vi "Periodic Tasks.vi"(8 "error in":errorcluster) -> ()   [LabVIEW 2019]
doc: "This VI runs in parallel to other tasks. It can contain as many user-defined periodic loops as you need. These can carry out PID or other sorts of timed response."
uses:
  <vilib>/Rock Robotics/Network Tables/NT Read Boolean.vi
  <vilib>/Rock Robotics/Network Tables/NT Write Number.vi
  <vilib>/Rock Robotics/Network Tables/NT Read Number.vi
  <vilib>/Rock Robotics/Network Tables/NT Write Boolean.vi
  <vilib>/Rock Robotics/WPI/Utilities/WPI_GetSetVariantRefNum.vi
  <vilib>/Rock Robotics/Network Tables/NT Write Numeric Array.vi
  <vilib>/Rock Robotics/WPI/RobotDrive/WPI_RobotDriveArcadeDrive_Standard(NoSaturation).vi
  <vilib>/express/express arith-compare/Formula/XNode/ExpressFormulaBlockNode.xnode
  <vilib>/Rock Robotics/Network Tables/NT Write String.vi
  <vilib>/Rock Robotics/Network Tables/NT Read String.vi
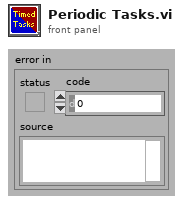
[diagram p1: front panel]
types:
  T1 = typedef "WPI_JoystickDevRef.ctl" = cluster{"Device":T2}
  T2 = typedef "WPI_JoystickDeviceEnum.ctl" = enum16{"USB 0", "USB 1", "USB 2", "USB 3", "USB 4", "USB 5"}
  T3 = typedef "WPI_RobotDriveDevRef.ctl" = cluster{"DevStatus":errorcluster, "Motors[]":T4[], "Square Inputs":bool, "Max Output":dbl}
  T4 = typedef "WPI_MotorControlDeviceRef.ctl" = cluster{"DeviceStatus":errorcluster, "Type":T5, "PWM":cluster{"PWM Channel":T6, "DeadBand":T7}, "CAN":cluster{"Device Number":u8, "SetOutput VI Ref":variant, "GetOutput VI Ref":variant, "Enable VI Ref":variant, "Disable VI Ref":variant, "Data":variant}, "Invert":bool, "DIO PWM":cluster{"PWM \"Enable\" Channel":T6, "DIOChannel":T8, "PWM Rate":dbl}}
  T5 = typedef "WPI_MotorControlType.ctl" = enum16{"PWM", "CAN", "DIO PWM"}
  T6 = typedef "FPGA_DIOPWMChannel.ctl" = enum8{"PWM 0", "PWM 1", "PWM 2", "PWM 3", "PWM 4", "PWM 5", "PWM 6", "PWM 7", "PWM 8", "PWM 9", "PWM MXP 0", "PWM MXP 1", "PWM MXP 2", "PWM MXP 3", "PWM MXP 4", "PWM MXP 5", "PWM MXP 6", "PWM MXP 7", "PWM MXP 8", "PWM MXP 9", "Invalid"}
  T7 = typedef "WPI_PWMDeadband.ctl" = cluster{"Name":string, "maxPositivePwm":i32, "minPositivePwm":i32, "centerPwm":i32, "maxNegativePwm":i32, "minNegativePwm":i32, "angularRange":u16}
  T8 = typedef "FPGA_DIOChannel.ctl" = enum8{"DIO 0", "DIO 1", "DIO 2", "DIO 3", "DIO 4", "DIO 5", "DIO 6", "DIO 7", "DIO 8", "DIO 9", "DIO MXP 0", "DIO MXP 1", "DIO MXP 2", "DIO MXP 3", "DIO MXP 4", "DIO MXP 5", "DIO MXP 6", "DIO MXP 7", "DIO MXP 8", "DIO MXP 9", "DIO MXP 10", "DIO MXP 11", "DIO MXP 12", "DIO MXP 13", "DIO MXP 14", "DIO MXP 15", "SPI Port CS1", "SPI Port CS2", "SPI Port CS3", "SPI Port MISO", "SPI Port MOSI", "Invalid"}
  T9 = cluster{"JoystickDevRef":T1, "RobotDriveDevRef":T3}
  T10 = typedef "Color Sensor V3 DevRef.ctl" = cluster{"I2CDevRef":T11}
  T11 = typedef "WPI_I2CDevRef.ctl" = cluster{"DevStatus":errorcluster, "Device Address":u8, "Handle":i32, "I2C Bus":T12}
  T12 = typedef "i2c_bus.ctl" = enum16{"I2C On-Board", "I2C MXP", "Invalid"}
  T13 = typedef "WPI_SwitchDevRef.ctl" = cluster{"DevStatus":errorcluster, "DIO Channel":T8, "CntIndex":T14, "Normally Closed":bool}
  T14 = typedef "FPGA_CounterCtrSystemIndex.ctl" = enum8{"Ctr 0", "Ctr 1", "Ctr 2", "Ctr 3", "Ctr 4", "Ctr 5", "Ctr 6", "Ctr 7", "Invalid"}
  T15 = typedef "WPI_ServoDeviceRef.ctl" = cluster{"DeviceStatus":errorcluster, "PWM Channel":T6, "DeadBand":T7}
  T16 = typedef "WPI_EncoderDevRef.ctl" = cluster{"DevStatus":errorcluster, "EncoderIndex":T17, "CounterIndex":T14, "DistancePerCount":dbl, "Decoding Type":T18}
  T17 = typedef "FPGA_EncoderIdx.ctl" = enum8{"Enc 0", "Enc 1", "Enc 2", "Enc 3", "Enc 4", "Enc 5", "Enc 6", "Enc 7", "Invalid"}
  T18 = typedef "WPI_EncoderType.ctl" = enum16{"1x", "2x", "4x"}
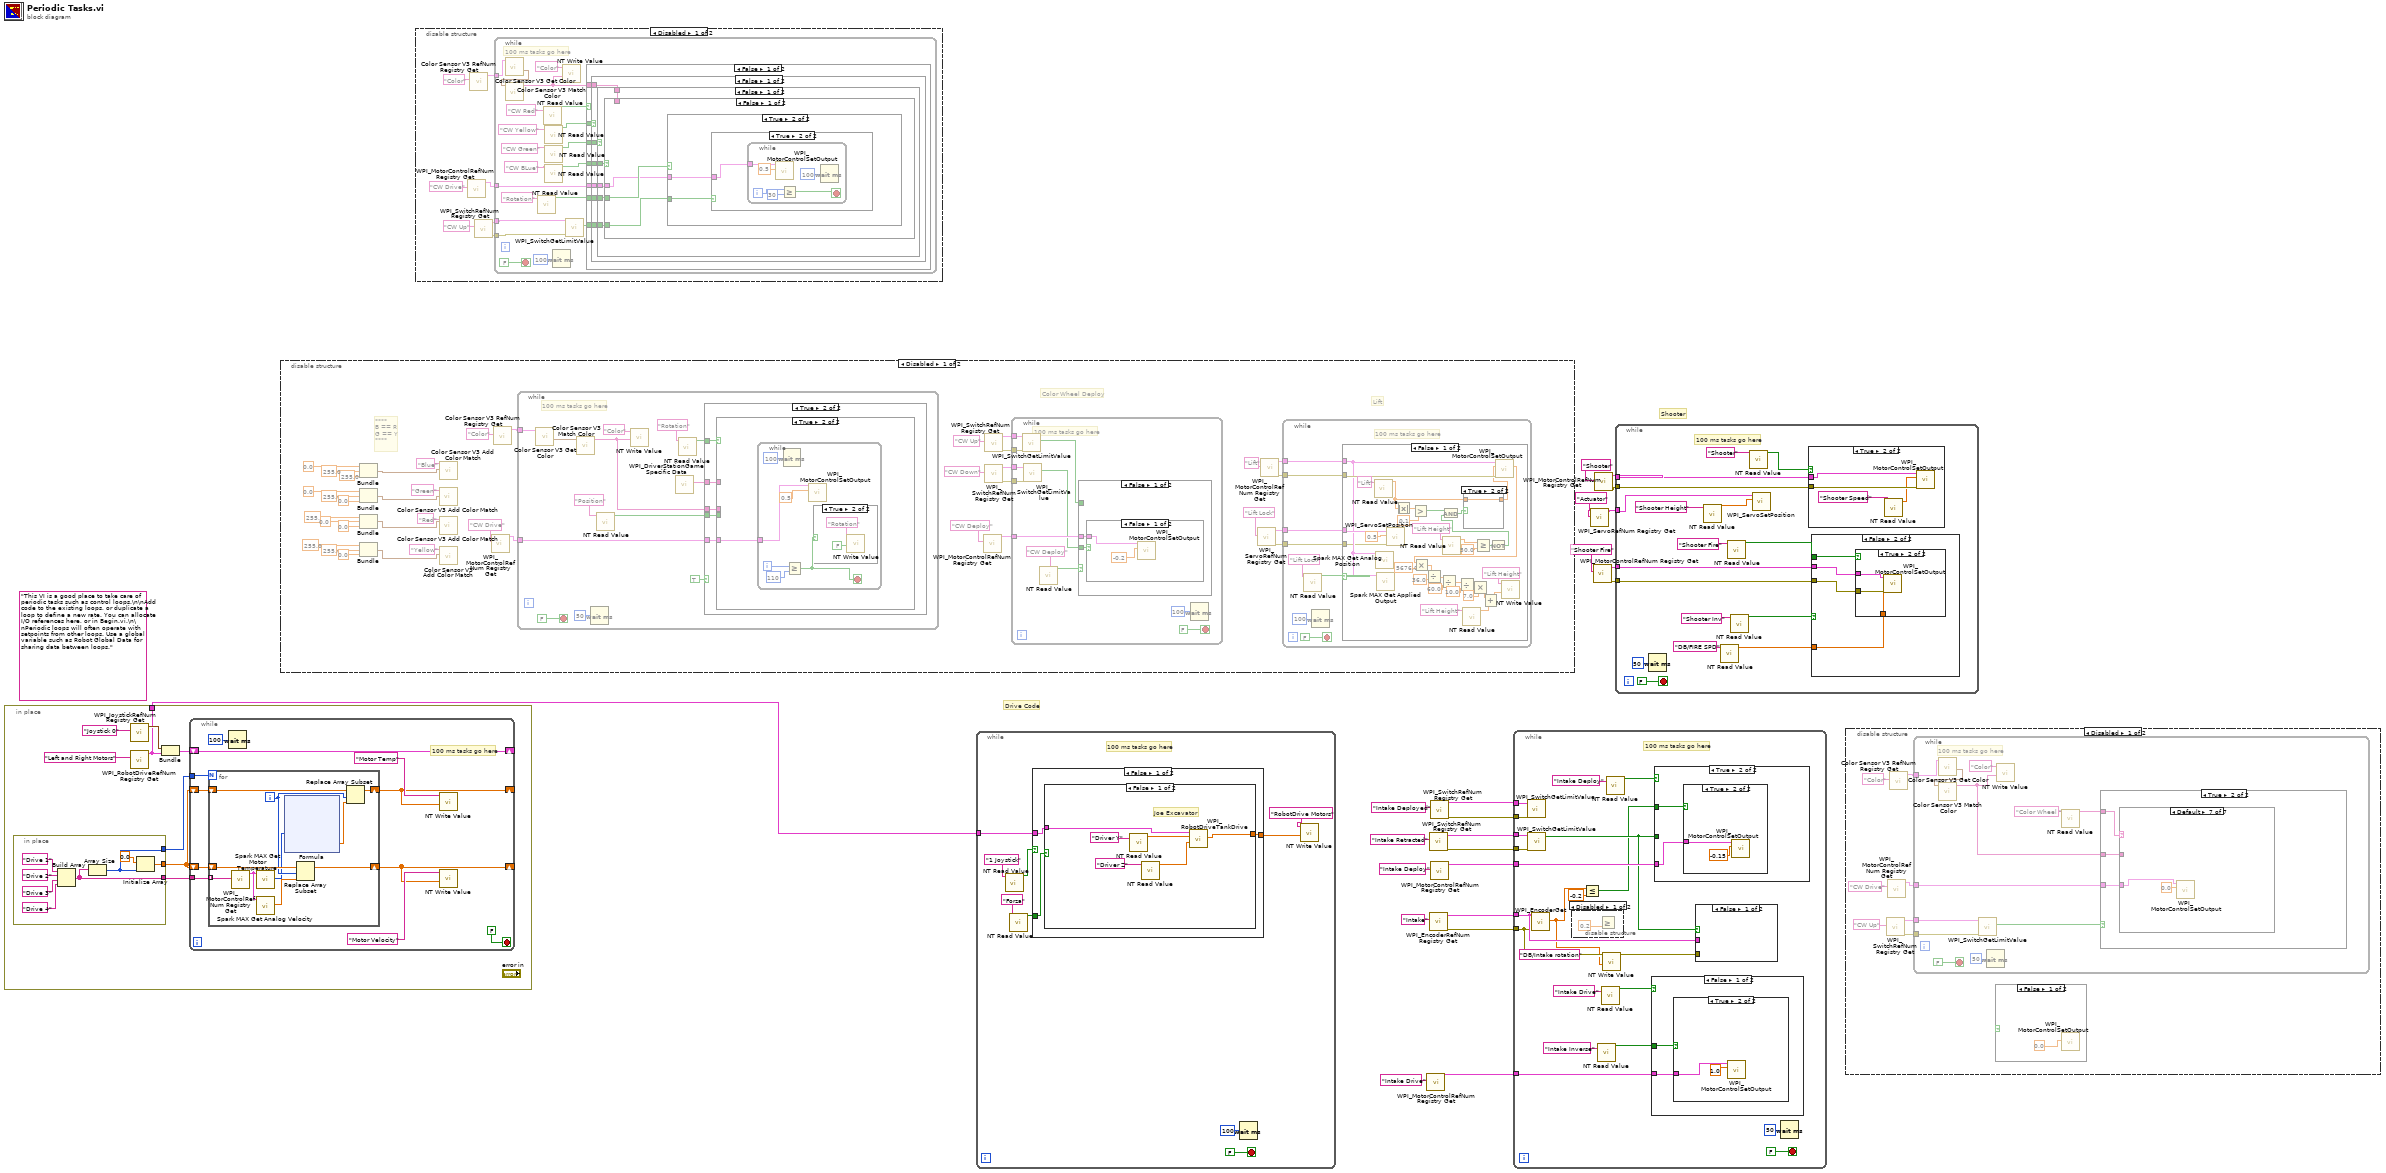
[diagram p0: block diagram]
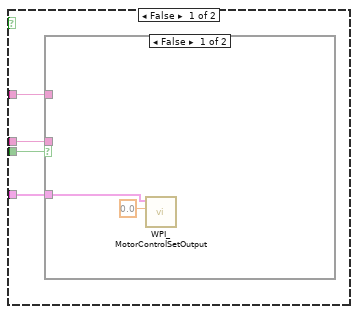
[diagram p3: hidden frame]
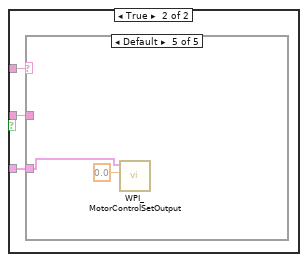
[diagram p4: hidden frame]
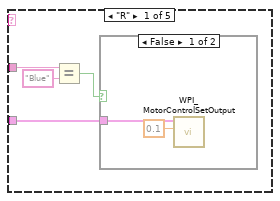
[diagram p5: hidden frame]
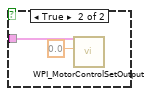
[diagram p6: hidden frame]
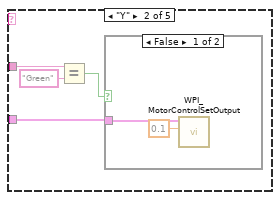
[diagram p7: hidden frame]
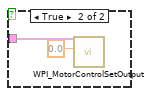
[diagram p8: hidden frame]
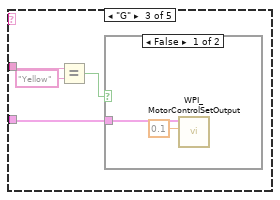
[diagram p9: hidden frame]
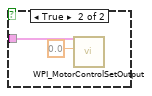
[diagram p10: hidden frame]
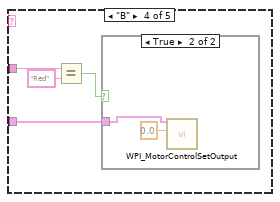
[diagram p11: hidden frame]
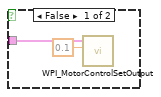
[diagram p12: hidden frame]
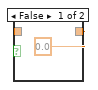
[diagram p14: hidden frame]
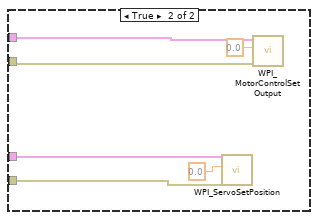
[diagram p15: hidden frame]
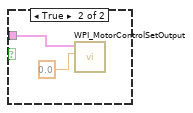
[diagram p16: hidden frame]
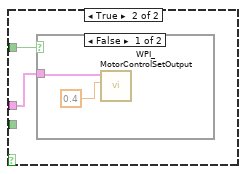
[diagram p17: hidden frame]
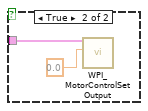
[diagram p18: hidden frame]
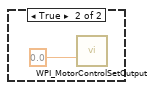
[diagram p20: hidden frame]
diagram:
  (unwired) "This VI is a good place to take care of periodic tasks such as control loops.\n\nAdd code to the existing loops, or duplicate a loop to define a new rate. You can allocate I/O references here, or in Begin.vi.\n\nPeriodic loops will often operate with setpoints from other loops. Use a global variable such as Robot Global Data for sharing data between loops."
  # "Shooter"
  # "Drive Code"
  n1 = in-place {
    in-place-border: [w23] -> w1
    n2 = in-place {
      in-place-border: [w34] -> w26
      in-place-border: [w33] -> w25
      in-place-border: [w31] -> w24
      n3 = Build Array("Drive 1", "Drive 2", "Drive 3", "Drive 4") -> (w34:string[])
      n4 = Array Size(array=w34) -> (size(s)=w33:i32)
      n5 = Initialize Array(0.0 ("element"), w33) -> (w31:dbl[])
    }
    n6 = call <vilib>:"WPI_JoystickRefNum Registry Get.vi"("refnum name"="Joystick 0") -> ("JoystickDevRef"=w28:T1)  [unwired: 1 in, 9 out]
    n7 = call <vilib>:"WPI_RobotDriveRefNum Registry Get.vi"("refnum name"="Left and Right Motors") -> ("RobotDriveDevRef"=w23:T3)  [unwired: 1 in, 9 out]
    n8 = Bundle("JoystickDevRef"=w28, "RobotDriveDevRef"=w23) -> (w27:T9)  [unwired: 1 out]
    n9 = while {
      shift-right: [w47] -> _
      shift-left: w27 -> [w47]
      tunnel: w26 -> [w44]
      tunnel: w25 -> [w43]
      shift-right: [w39] -> _
      shift-left: w24 -> [w42]
      shift-right: [w40] -> _
      shift-left: w24 -> [w41]
      stop <- FALSE stop-if-true
      # "100 ms tasks go here"
      n10 = for {
        N: w43 -> [_]
        tunnel: w44 -> [w58] mode=indexing
        shift-right: [w55] -> w40
        shift-left: w41 -> [w56]
        shift-right: [w53] -> w39
        shift-left: w42 -> [w57]
        i -> [w52]
        n11 = call <vilib>:"WPI_MotorControlRefNum Registry Get.vi"("refnum name"=w58) -> ("MotorControlDevRef"=w59:T4)  [unwired: 9 in, 1 out]
        n12 = call <vilib>:"Spark MAX Get Motor Temperature.vi"("MotorControlDevRef in"=w59) -> ("Motor Temperature"=w51:u8)  [unwired: 7 in, 3 out]
        n13 = call <vilib>:"Spark MAX Get Analog Velocity.vi"("MotorControlDevRef in"=w59) -> ("Analog Velocity"=w54:dbl)  [unwired: 7 in, 3 out]
        n14 = xnode "Formula"("degC"=w51) -> ("Result"=w50:dbl)  [unwired: 1 in, 1 out]
        n15 = Replace Array Subset(array=w56, new element=w54, index=w52) -> (w55:dbl[])
        n16 = Replace Array Subset(array=w57, new element=w50, index=w52) -> (w53:dbl[])
      }
      n17 = Wait (ms)(milliseconds to wait=u32 100) -> ()  [unwired: 1 out]
      n18 = call-poly <vilib>:"NT Write Value.vi"("Numeric Array"=w39, "Name"="Motor Temp") -> ()  [unwired: 9 in, 1 out]
      n19 = call-poly <vilib>:"NT Write Value.vi"("Numeric Array"=w40, "Name"="Motor Velocity") -> ()  [unwired: 9 in, 1 out]
    }
  }
  n20 = disable-structure shown="Disabled" {
    frame Disabled {
      # "Lift"
      # "****\nB == R\nG == Y\n****"
      # "Color Wheel Deploy"
      n21 = Bundle(0.0, 255.0, 255.0) -> (w99:cluster{dbl, dbl, dbl})  [unwired: 1 in]
      n22 = Bundle(0.0, 255.0, 0.0) -> (w94:cluster{dbl, dbl, dbl})  [unwired: 1 in]
      n23 = Bundle(255.0, 0.0, 0.0) -> (w87:cluster{dbl, dbl, dbl})  [unwired: 1 in]
      n24 = Bundle(255.0, 255.0, 0.0) -> (w86:cluster{dbl, dbl, dbl})  [unwired: 1 in]
      n25 = call <vilib>:"Color Sensor V3 Add Color Match.vi"("Color"=w94, "Name"="Green") -> ()  [unwired: 10 in]
      n26 = call <vilib>:"Color Sensor V3 Add Color Match.vi"("Color"=w87, "Name"="Red") -> ()  [unwired: 10 in]
      n27 = call <vilib>:"Color Sensor V3 Add Color Match.vi"("Color"=w99, "Name"="Blue") -> ()  [unwired: 10 in]
      n28 = call <vilib>:"Color Sensor V3 Add Color Match.vi"("Color"=w86, "Name"="Yellow") -> ()  [unwired: 10 in]
      n29 = call <vilib>:"WPI_MotorControlRefNum Registry Get.vi"("refnum name"="CW Drive") -> ("MotorControlDevRef"=w68:T4)  [unwired: 9 in, 1 out]
      n30 = call <vilib>:"Color Sensor V3 RefNum Registry Get.vi"("refnum name"="Color") -> ("ColorSensorDevRef"=w70:T10)  [unwired: 9 in, 1 out]
      n31 = while {
        tunnel: w70 -> [w116]
        tunnel: w68 -> [w112]
        stop <- FALSE stop-if-true
        # "100 ms tasks go here"
        n32 = call <vilib>:"Color Sensor V3 Get Color.vi"("ColorSensorDevRef"=w116) -> ("Normalized Color"=w115:cluster{"R":dbl, "G":dbl, "B":dbl})  [unwired: 7 in, 3 out]
        n33 = call <vilib>:"Color Sensor V3 Match Color.vi"("Measured Color"=w115) -> ("Matched Color Name"=w113:string)  [unwired: 8 in, 2 out]
        n34 = Wait (ms)(milliseconds to wait=u32 50) -> ()  [unwired: 1 out]
        n35 = call-poly <vilib>:"NT Read Value.vi"("Name"="Position") -> ("Boolean"=w106:bool)  [unwired: 9 in, 1 out]
        n36 = call-poly <vilib>:"NT Write Value.vi"("String"=w113, "Name"="Color") -> ()  [unwired: 9 in, 1 out]
        n37 = call <vilib>:"WPI_DriverStationGame Specific Data.vi"() -> ("Game Specific Data"=w111:string)  [unwired: 11 in]
        n38 = call-poly <vilib>:"NT Read Value.vi"("Name"="Rotation") -> ("Boolean"=w109:bool)  [unwired: 9 in, 1 out]
        n39 = case shown="True" TRUE {
          tunnel: w111 -> [_ w122]
          tunnel: w113 -> [_ w121]
          tunnel: w112 -> [_ w120]
          tunnel: w109 -> [_ w123]
          tunnel: w106 -> [_ w119]
          frame False {
          }
          frame True {
            n40 = case shown="True" w123 {
              tunnel: w122 -> [w127 _]
              tunnel: w121 -> [w126 _]
              tunnel: w120 -> [w125 w167]
              tunnel: w119 -> [w124 _]
              frame False {
                n41 = case shown="False" w124 {
                  tunnel: w127 -> [_ w132]
                  tunnel: w126 -> [_ w131]
                  tunnel: w125 -> [w128 w130]
                  frame False {
                    n42 = call <vilib>:"WPI_MotorControlSetOutput.vi"("Output"=0.0, "MotorControlDevRef"=w128) -> ()  [unwired: 7 in, 3 out]
                  }
                  frame True {
                    n43 = case shown="Default" w132 {
                      tunnel: w131 -> [w136 w141 w150 w158 _]
                      tunnel: w130 -> [w134 w142 w149 w157 w165]
                      frame "R" {
                        n44 = Equal?(x=w136, y="Blue") -> (x = y?=w135:bool)
                        n45 = case shown="False" w135 {
                          tunnel: w134 -> [w138 w140]
                          frame False {
                            n46 = call <vilib>:"WPI_MotorControlSetOutput.vi"("Output"=0.1, "MotorControlDevRef"=w138) -> ()  [unwired: 7 in, 3 out]
                          }
                          frame True {
                            n47 = call <vilib>:"WPI_MotorControlSetOutput.vi"("Output"=0.0, "MotorControlDevRef"=w140) -> ()  [unwired: 7 in, 3 out]
                          }
                        }
                      }
                      frame "Y" {
                        n48 = Equal?(x=w141, y="Green") -> (x = y?=w144:bool)
                        n49 = case shown="False" w144 {
                          tunnel: w142 -> [w146 w148]
                          frame False {
                            n50 = call <vilib>:"WPI_MotorControlSetOutput.vi"("Output"=0.1, "MotorControlDevRef"=w146) -> ()  [unwired: 7 in, 3 out]
                          }
                          frame True {
                            n51 = call <vilib>:"WPI_MotorControlSetOutput.vi"("Output"=0.0, "MotorControlDevRef"=w148) -> ()  [unwired: 7 in, 3 out]
                          }
                        }
                      }
                      frame "G" {
                        n52 = Equal?(x=w150, y="Yellow") -> (x = y?=w152:bool)
                        n53 = case shown="False" w152 {
                          tunnel: w149 -> [w154 w156]
                          frame False {
                            n54 = call <vilib>:"WPI_MotorControlSetOutput.vi"("Output"=0.1, "MotorControlDevRef"=w154) -> ()  [unwired: 7 in, 3 out]
                          }
                          frame True {
                            n55 = call <vilib>:"WPI_MotorControlSetOutput.vi"("Output"=0.0, "MotorControlDevRef"=w156) -> ()  [unwired: 7 in, 3 out]
                          }
                        }
                      }
                      frame "B" {
                        n56 = Equal?(x=w158, y="Red") -> (x = y?=w160:bool)
                        n57 = case shown="True" w160 {
                          tunnel: w157 -> [w161 w163]
                          frame False {
                            n58 = call <vilib>:"WPI_MotorControlSetOutput.vi"("Output"=0.1, "MotorControlDevRef"=w161) -> ()  [unwired: 7 in, 3 out]
                          }
                          frame True {
                            n59 = call <vilib>:"WPI_MotorControlSetOutput.vi"("Output"=0.0, "MotorControlDevRef"=w163) -> ()  [unwired: 7 in, 3 out]
                          }
                        }
                      }
                      frame Default {
                        n60 = call <vilib>:"WPI_MotorControlSetOutput.vi"("Output"=0.0, "MotorControlDevRef"=w165) -> ()  [unwired: 7 in, 3 out]
                      }
                    }
                  }
                }
              }
              frame True {
                n61 = while {
                  tunnel: w167 -> [w168]
                  i -> [w172]
                  stop <- w170 stop-if-true
                  n62 = Wait (ms)(milliseconds to wait=u32 100) -> ()  [unwired: 1 out]
                  n63 = Greater Or Equal?(x=w172, y=110) -> (x >= y?=w170:bool)
                  n64 = call <vilib>:"WPI_MotorControlSetOutput.vi"("Output"=0.5, "MotorControlDevRef"=w168) -> ()  [unwired: 7 in, 3 out]
                  n65 = case shown="True" w170 {
                    frame False {
                    }
                    frame True {
                      n66 = call-poly <vilib>:"NT Write Value.vi"("Boolean"=FALSE, "Name"="Rotation") -> ()  [unwired: 9 in, 1 out]
                    }
                  }
                }
              }
            }
          }
        }
      }
      n67 = call <vilib>:"WPI_MotorControlRefNum Registry Get.vi"("refnum name"="CW Deploy") -> ("MotorControlDevRef"=w82:T4)  [unwired: 9 in, 1 out]
      n68 = call <vilib>:"WPI_SwitchRefNum Registry Get.vi"("refnum name"="CW Up") -> ("error out"=w74:errorcluster, "SwitchDevRef"=w73:T13)  [unwired: 9 in]
      n69 = call <vilib>:"WPI_SwitchRefNum Registry Get.vi"("refnum name"="CW Down") -> ("error out"=w76:errorcluster, "SwitchDevRef"=w75:T13)  [unwired: 9 in]
      n70 = while {
        tunnel: w82 -> [w230]
        tunnel: w76 -> [w229]
        tunnel: w75 -> [w228]
        tunnel: w74 -> [w226]
        tunnel: w73 -> [w225]
        stop <- FALSE stop-if-true
        # "100 ms tasks go here"
        n71 = call <vilib>:"WPI_SwitchGetLimitValue.vi"("error in (no error)"=w226, "SwitchDevRef"=w225) -> ("Switch Pressed"=w224:bool)  [unwired: 7 in, 2 out]
        n72 = call <vilib>:"WPI_SwitchGetLimitValue.vi"("error in (no error)"=w229, "SwitchDevRef"=w228) -> ("Switch Pressed"=w227:bool)  [unwired: 7 in, 2 out]
        n73 = call-poly <vilib>:"NT Read Value.vi"("Name"="CW Deploy") -> ("Boolean"=w231:bool)  [unwired: 9 in, 1 out]
        n74 = case shown="False" w231 {
          tunnel: w230 -> [w236 w241]
          tunnel: w227 -> [w235 _]
          tunnel: w224 -> [_ w242]
          frame False {
            n75 = case shown="False" w235 {
              tunnel: w236 -> [w237 w240]
              frame False {
                n76 = call <vilib>:"WPI_MotorControlSetOutput.vi"("Output"=-0.2 ("Motor Output"), "MotorControlDevRef"=w237) -> ()  [unwired: 7 in, 3 out]
              }
              frame True {
                n77 = call <vilib>:"WPI_MotorControlSetOutput.vi"("Output"=0.0 ("Motor Output"), "MotorControlDevRef"=w240) -> ()  [unwired: 7 in, 3 out]
              }
            }
          }
          frame True {
            n78 = case shown="False" w242 {
              tunnel: w241 -> [w243 w246]
              frame False {
                n79 = call <vilib>:"WPI_MotorControlSetOutput.vi"("Output"=0.4 ("Motor Output"), "MotorControlDevRef"=w243) -> ()  [unwired: 7 in, 3 out]
              }
              frame True {
                n80 = call <vilib>:"WPI_MotorControlSetOutput.vi"("Output"=0.0 ("Motor Output"), "MotorControlDevRef"=w246) -> ()  [unwired: 7 in, 3 out]
              }
            }
          }
        }
        n81 = Wait (ms)(milliseconds to wait=u32 100) -> ()  [unwired: 1 out]
      }
      n82 = call <vilib>:"WPI_ServoRefNum Registry Get.vi"("refnum name"="Lift Lock") -> ("error out"=w72:errorcluster, "ServoDeviceRef"=w77:T15)  [unwired: 9 in]
      n83 = call <vilib>:"WPI_MotorControlRefNum Registry Get.vi"("refnum name"="Lift") -> ("error out"=w79:errorcluster, "MotorControlDevRef"=w80:T4)  [unwired: 9 in]
      n84 = while {
        tunnel: w80 -> [w176]
        tunnel: w79 -> [w177]
        tunnel: w77 -> [w181]
        tunnel: w72 -> [w178]
        stop <- FALSE stop-if-true
        # "100 ms tasks go here"
        n85 = call-poly <vilib>:"NT Read Value.vi"("Name"="Lift Lock") -> ("Boolean"=w179:bool)  [unwired: 9 in, 1 out]
        n86 = Wait (ms)(milliseconds to wait=u32 100) -> ()  [unwired: 1 out]
        n87 = case shown="False" w179 {
          tunnel: w181 -> [w215 w223]
          tunnel: w178 -> [w204 w222]
          tunnel: w177 -> [w213 w219]
          tunnel: w176 -> [w207 w220]
          frame False {
            n88 = call-poly <vilib>:"NT Read Value.vi"("Name"="Lift") -> ("Numeric"=w208:dbl)  [unwired: 9 in, 1 out]
            n89 = call <vilib>:"Spark MAX Get Analog Position.vi"("MotorControlDevRef in"=w207) -> ()  [unwired: 7 in, 4 out]
            n90 = call <vilib>:"Spark MAX Get Applied Output.vi"("MotorControlDevRef in"=w207) -> ()  [unwired: 7 in, 4 out]
            n91 = call <vilib>:"WPI_ServoSetPosition.vi"("error in (no error)"=w204, "Position"=0.5, "ServoDeviceRef"=w215) -> ()  [unwired: 7 in, 2 out]
            n92 = Absolute Value(x=w208) -> (abs(x)=w211:dbl)
            n93 = Greater?(x=w211, y=0.1) -> (0:w187:bool)
            n94 = call-poly <vilib>:"NT Read Value.vi"("Name"="Lift Height") -> ("Numeric"=w189:dbl)  [unwired: 9 in, 1 out]
            n95 = call-poly <vilib>:"NT Read Value.vi"("Name"="Lift Height") -> ("Numeric"=w192:dbl)  [unwired: 9 in, 1 out]
            n96 = Greater Or Equal?(x=w189, y=50.0) -> (x >= y?=w185:bool)
            n97 = Not(x=w185) -> (.not. x?=w184:bool)
            n98 = And(x=w187, y=w184) -> (x .and. y?=w186:bool)
            n99 = case shown="True" w186 {
              tunnel: [0.0 w217] -> w209
              tunnel: w208 -> [_ w217]
              frame False {
              }
              frame True {
              }
            }
            n100 = call <vilib>:"WPI_MotorControlSetOutput.vi"("error in (no error)"=w213, "Output"=w209, "MotorControlDevRef"=w207) -> ("Motor Output"=w196:dbl)  [unwired: 6 in, 2 out]
            n101 = Multiply(x=w196, y=5676.0) -> (x*y=w198:dbl)
            n102 = Divide(x=w198, y=36.0) -> (x/y=w201:dbl)
            n103 = Divide(x=w201, y=60.0) -> (x/y=w202:dbl)
            n104 = Divide(x=w202, y=10.0) -> (x/y=w200:dbl)
            n105 = Multiply(x=w200, y=7.0) -> (x*y=w191:dbl)
            n106 = Add(x=w191, y=w192) -> (x+y=w193:dbl)
            n107 = call-poly <vilib>:"NT Write Value.vi"("Numeric"=w193, "Name"="Lift Height") -> ()  [unwired: 9 in, 1 out]
          }
          frame True {
            n108 = call <vilib>:"WPI_ServoSetPosition.vi"("error in (no error)"=w222, "Position"=0.0, "ServoDeviceRef"=w223) -> ()  [unwired: 7 in, 2 out]
            n109 = call <vilib>:"WPI_MotorControlSetOutput.vi"("error in (no error)"=w219, "Output"=0.0, "MotorControlDevRef"=w220) -> ()  [unwired: 6 in, 3 out]
          }
        }
      }
    }
    frame Enabled {
    }
  }
  n110 = disable-structure shown="Disabled" {
    frame Disabled {
      n111 = call <vilib>:"WPI_MotorControlRefNum Registry Get.vi"("refnum name"="CW Drive") -> ("MotorControlDevRef"=w250:T4)  [unwired: 9 in, 1 out]
      n112 = call <vilib>:"Color Sensor V3 RefNum Registry Get.vi"("refnum name"="Color") -> ("ColorSensorDevRef"=w252:T10)  [unwired: 9 in, 1 out]
      n113 = call <vilib>:"WPI_SwitchRefNum Registry Get.vi"("refnum name"="CW Up") -> ("error out"=w247:errorcluster, "SwitchDevRef"=w248:T13)  [unwired: 9 in]
      n114 = while {
        tunnel: w252 -> [w271]
        tunnel: w250 -> [w261]
        tunnel: w248 -> [w258]
        tunnel: w247 -> [w257]
        stop <- FALSE stop-if-true
        # "100 ms tasks go here"
        n115 = call <vilib>:"Color Sensor V3 Get Color.vi"("ColorSensorDevRef"=w271) -> ("Normalized Color"=w270:cluster{"R":dbl, "G":dbl, "B":dbl})  [unwired: 7 in, 3 out]
        n116 = call <vilib>:"Color Sensor V3 Match Color.vi"("Measured Color"=w270) -> ("Matched Color Name"=w255:string)  [unwired: 8 in, 2 out]
        n117 = call-poly <vilib>:"NT Read Value.vi"("Name"="Rotation") -> ("Boolean"=w259:bool)  [unwired: 9 in, 1 out]
        n118 = call-poly <vilib>:"NT Read Value.vi"("Name"="CW Red") -> ("Boolean"=w266:bool)  [unwired: 9 in, 1 out]
        n119 = call-poly <vilib>:"NT Read Value.vi"("Name"="CW Yellow") -> ("Boolean"=w265:bool)  [unwired: 9 in, 1 out]
        n120 = call-poly <vilib>:"NT Read Value.vi"("Name"="CW BLue") -> ("Boolean"=w262:bool)  [unwired: 9 in, 1 out]
        n121 = call-poly <vilib>:"NT Read Value.vi"("Name"="CW Green") -> ("Boolean"=w264:bool)  [unwired: 9 in, 1 out]
        n122 = Wait (ms)(milliseconds to wait=u32 100) -> ()  [unwired: 1 out]
        n123 = call-poly <vilib>:"NT Write Value.vi"("String"=w255, "Name"="Color") -> ()  [unwired: 9 in, 1 out]
        n124 = call <vilib>:"WPI_SwitchGetLimitValue.vi"("error in (no error)"=w257, "SwitchDevRef"=w258) -> ("Switch Pressed"=w256:bool)  [unwired: 7 in, 2 out]
        n125 = case shown="False" w266 {
          tunnel: w265 -> [w280 _]
          tunnel: w264 -> [w279 _]
          tunnel: w262 -> [w278 _]
          tunnel: w255 -> [w277 w334]
          tunnel: w261 -> [w276 w332]
          tunnel: w259 -> [w275 _]
          tunnel: w256 -> [w274 _]
          frame False {
            n126 = case shown="False" w280 {
              tunnel: w279 -> [w286 _]
              tunnel: w278 -> [w285 _]
              tunnel: w277 -> [w284 w327]
              tunnel: w276 -> [w283 w324]
              tunnel: w275 -> [w282 _]
              tunnel: w274 -> [w281 _]
              frame False {
                n127 = case shown="False" w286 {
                  tunnel: w285 -> [w291 _]
                  tunnel: w284 -> [w290 w319]
                  tunnel: w283 -> [w289 w316]
                  tunnel: w282 -> [w288 _]
                  tunnel: w281 -> [w287 _]
                  frame False {
                    n128 = case shown="False" w291 {
                      tunnel: w290 -> [_ w309]
                      tunnel: w289 -> [w293 w308]
                      tunnel: w288 -> [w294 _]
                      tunnel: w287 -> [w292 _]
                      frame False {
                        n129 = case shown="True" w294 {
                          tunnel: w293 -> [w295 w298]
                          tunnel: w292 -> [_ w297]
                          frame False {
                            n130 = call <vilib>:"WPI_MotorControlSetOutput.vi"("Output"=0.0, "MotorControlDevRef"=w295) -> ()  [unwired: 7 in, 3 out]
                          }
                          frame True {
                            n131 = case shown="True" w297 {
                              tunnel: w298 -> [w299 w301]
                              frame False {
                                n132 = call <vilib>:"WPI_MotorControlSetOutput.vi"("Output"=0.0, "MotorControlDevRef"=w299) -> ()  [unwired: 7 in, 3 out]
                              }
                              frame True {
                                n133 = while {
                                tunnel: w301 -> [w306]
                                i -> [w304]
                                stop <- w302 stop-if-true
                                n134 = call <vilib>:"WPI_MotorControlSetOutput.vi"("Output"=0.5, "MotorControlDevRef"=w306) -> ()  [unwired: 7 in, 3 out]
                                n135 = Greater Or Equal?(x=w304, y=30) -> (x >= y?=w302:bool)
                                n136 = Wait (ms)(milliseconds to wait=u32 100) -> ()  [unwired: 1 out]
                                }
                              }
                            }
                          }
                        }
                      }
                      frame True {
                        n137 = Equal?(x=w309, y="Red") -> (x = y?=w310:bool)
                        n138 = case shown="False" w310 {
                          tunnel: w308 -> [w312 w314]
                          frame False {
                            n139 = call <vilib>:"WPI_MotorControlSetOutput.vi"("Output"=0.1, "MotorControlDevRef"=w312) -> ()  [unwired: 7 in, 3 out]
                          }
                          frame True {
                            n140 = call <vilib>:"WPI_MotorControlSetOutput.vi"("Output"=0.0, "MotorControlDevRef"=w314) -> ()  [unwired: 7 in, 3 out]
                          }
                        }
                      }
                    }
                  }
                  frame True {
                    n141 = Equal?(x=w319, y="Yellow") -> (x = y?=w317:bool)
                    n142 = case shown="True" w317 {
                      tunnel: w316 -> [w320 w322]
                      frame False {
                        n143 = call <vilib>:"WPI_MotorControlSetOutput.vi"("Output"=0.1, "MotorControlDevRef"=w320) -> ()  [unwired: 7 in, 3 out]
                      }
                      frame True {
                        n144 = call <vilib>:"WPI_MotorControlSetOutput.vi"("Output"=0.0, "MotorControlDevRef"=w322) -> ()  [unwired: 7 in, 3 out]
                      }
                    }
                  }
                }
              }
              frame True {
                n145 = Equal?(x=w327, y="Green") -> (x = y?=w326:bool)
                n146 = case shown="True" w326 {
                  tunnel: w324 -> [w328 w330]
                  frame False {
                    n147 = call <vilib>:"WPI_MotorControlSetOutput.vi"("Output"=0.1, "MotorControlDevRef"=w328) -> ()  [unwired: 7 in, 3 out]
                  }
                  frame True {
                    n148 = call <vilib>:"WPI_MotorControlSetOutput.vi"("Output"=0.0, "MotorControlDevRef"=w330) -> ()  [unwired: 7 in, 3 out]
                  }
                }
              }
            }
          }
          frame True {
            n149 = Equal?(x=w334, y="Blue") -> (x = y?=w335:bool)
            n150 = case shown="True" w335 {
              tunnel: w332 -> [w336 w338]
              frame False {
                n151 = call <vilib>:"WPI_MotorControlSetOutput.vi"("Output"=0.1, "MotorControlDevRef"=w336) -> ()  [unwired: 7 in, 3 out]
              }
              frame True {
                n152 = call <vilib>:"WPI_MotorControlSetOutput.vi"("Output"=0.0, "MotorControlDevRef"=w338) -> ()  [unwired: 7 in, 3 out]
              }
            }
          }
        }
      }
    }
    frame Enabled {
    }
  }
  n153 = while {
    tunnel: w1 -> [w346]
    stop <- FALSE stop-if-true
    # "100 ms tasks go here"
    n154 = call-poly <vilib>:"NT Read Value.vi"("Name"="1 Joystick") -> ("Boolean"=w344:bool)  [unwired: 9 in, 1 out]
    n155 = call-poly <vilib>:"NT Read Value.vi"("Name"="Forza") -> ("Boolean"=w340:bool)  [unwired: 9 in, 1 out]
    n156 = case shown="False" w344 {
      tunnel: w346 -> [w351 w365]
      tunnel: [w350 w364] -> w343
      tunnel: w340 -> [w349 _]
      frame False {
        n157 = case shown="False" w349 {
          tunnel: w351 -> [w352 w359]
          tunnel: [w355 w358] -> w350
          frame False {
            # "Joe Excavator"
            n158 = call-poly <vilib>:"NT Read Value.vi"("Name"="Driver Y") -> ("Numeric"=w354:dbl)  [unwired: 9 in, 1 out]
            n159 = call-poly <vilib>:"NT Read Value.vi"("Name"="Driver Z") -> ("Numeric"=w353:dbl)  [unwired: 9 in, 1 out]
            n160 = call <vilib>:"WPI_RobotDriveTankDrive.vi"("Right axis value"=w353, "Left axis value"=w354, "RobotDriveDevRef"=w352) -> ("Motor Values"=w355:dbl[])  [unwired: 6 in, 2 out]
          }
          frame True {
            # "Nathan Forza"
            n161 = call-poly <vilib>:"NT Read Value.vi"("Name"="Driver Y") -> ("Numeric"=w361:dbl)  [unwired: 9 in, 1 out]
            n162 = call-poly <vilib>:"NT Read Value.vi"("Name"="Driver Z") -> ("Numeric"=w360:dbl)  [unwired: 9 in, 1 out]
            n163 = call-poly <vilib>:"WPI_RobotDriveArcadeDrive.vi"("Y axis value"=w360, "X axis value"=w361, "RobotDriveDevRef"=w359) -> ("Motor Values"=w358:dbl[])  [unwired: 6 in, 2 out]
          }
        }
      }
      frame True {
        n164 = call-poly <vilib>:"NT Read Value.vi"("Name"="Driver Y") -> ("Numeric"=w367:dbl)  [unwired: 9 in, 1 out]
        n165 = call-poly <vilib>:"NT Read Value.vi"("Name"="Driver Z") -> ("Numeric"=w366:dbl)  [unwired: 9 in, 1 out]
        n166 = call-poly <vilib>:"WPI_RobotDriveArcadeDrive.vi"("Y axis value"=w366, "X axis value"=w367, "RobotDriveDevRef"=w365) -> ("Motor Values"=w364:dbl[])  [unwired: 6 in, 2 out]
      }
    }
    n167 = Wait (ms)(milliseconds to wait=u32 100) -> ()  [unwired: 1 out]
    n168 = call-poly <vilib>:"NT Write Value.vi"("Numeric Array"=w343, "Name"="RobotDrive Motors") -> ()  [unwired: 9 in, 1 out]
  }
  n169 = call <vilib>:"WPI_MotorControlRefNum Registry Get.vi"("refnum name"="Intake Drive") -> ("MotorControlDevRef"=w19:T4)  [unwired: 9 in, 1 out]
  n170 = call <vilib>:"WPI_SwitchRefNum Registry Get.vi"("refnum name"="Intake Retracted") -> ("error out"=w6:errorcluster, "SwitchDevRef"=w7:T13)  [unwired: 9 in]
  n171 = call <vilib>:"WPI_EncoderRefNum Registry Get.vi"("refnum name"="Intake") -> ("error out"=w5:errorcluster, "EncoderDevRef"=w4:T16)  [unwired: 9 in]
  n172 = call <vilib>:"WPI_SwitchRefNum Registry Get.vi"("refnum name"="Intake Deployed") -> ("error out"=w10:errorcluster, "SwitchDevRef"=w11:T13)  [unwired: 9 in]
  n173 = call <vilib>:"WPI_MotorControlRefNum Registry Get.vi"("refnum name"="Intake Deploy") -> ("MotorControlDevRef"=w21:T4)  [unwired: 9 in, 1 out]
  n174 = while {
    tunnel: w21 -> [w386]
    tunnel: w19 -> [w383]
    tunnel: w11 -> [w380]
    tunnel: w10 -> [w379]
    tunnel: w7 -> [w378]
    tunnel: w6 -> [w377]
    tunnel: w5 -> [w374]
    tunnel: w4 -> [w375]
    stop <- FALSE stop-if-true
    # "100 ms tasks go here"
    n175 = call <vilib>:"WPI_SwitchGetLimitValue.vi"("error in (no error)"=w379, "SwitchDevRef"=w380) -> ()  [unwired: 7 in, 3 out]
    n176 = call <vilib>:"WPI_SwitchGetLimitValue.vi"("error in (no error)"=w377, "SwitchDevRef"=w378) -> ("Switch Pressed"=w376:bool)  [unwired: 7 in, 2 out]
    n177 = call <vilib>:"WPI_EncoderGet.vi"("error in (no error)"=w374, "EncoderDevRef"=w375) -> ("Distance"=w370:dbl)  [unwired: 4 in, 5 out]
    n178 = disable-structure shown="Disabled" {
      frame Disabled {
        n179 = Greater Or Equal?(y=0.2) -> ()  [unwired: 1 in, 1 out]
      }
      frame Enabled {
      }
    }
    n180 = Less Or Equal?(x=w370, y=-0.2) -> (x <= y?=w372:bool)
    n181 = call-poly <vilib>:"NT Read Value.vi"("Name"="Intake Inverse") -> ("Boolean"=w381:bool)  [unwired: 9 in, 1 out]
    n182 = call-poly <vilib>:"NT Read Value.vi"("Name"="Intake Drive") -> ("Boolean"=w385:bool)  [unwired: 9 in, 1 out]
    n183 = call-poly <vilib>:"NT Write Value.vi"("Numeric"=w370, "Name"="DB/Intake rotation") -> ()  [unwired: 9 in, 1 out]
    n184 = call-poly <vilib>:"NT Read Value.vi"("Name"="Intake Deploy") -> ("Boolean"=w388:bool)  [unwired: 9 in, 1 out]
    n185 = case shown="False" w385 {
      tunnel: w383 -> [w394 w400]
      tunnel: w381 -> [w395 _]
      frame False {
        n186 = case shown="True" w395 {
          tunnel: w394 -> [w396 w398]
          frame False {
            n187 = call <vilib>:"WPI_MotorControlSetOutput.vi"("Output"=0.0, "MotorControlDevRef"=w396) -> ()  [unwired: 7 in, 3 out]
          }
          frame True {
            n188 = call <vilib>:"WPI_MotorControlSetOutput.vi"("Output"=1.0, "MotorControlDevRef"=w398) -> ()  [unwired: 7 in, 3 out]
          }
        }
      }
      frame True {
        n189 = call <vilib>:"WPI_MotorControlSetOutput.vi"("Output"=-1.0, "MotorControlDevRef"=w400) -> ()  [unwired: 7 in, 3 out]
      }
    }
    n190 = case shown="True" w388 {
      tunnel: w386 -> [w402 w405]
      tunnel: w376 -> [_ _]
      tunnel: w372 -> [_ w404]
      frame False {
        n191 = call <vilib>:"WPI_MotorControlSetOutput.vi"("Output"=0.0, "MotorControlDevRef"=w402) -> ()  [unwired: 7 in, 3 out]
      }
      frame True {
        n192 = case shown="True" w404 {
          tunnel: w405 -> [w406 w408]
          frame False {
            n193 = call <vilib>:"WPI_MotorControlSetOutput.vi"("Output"=-1.0, "MotorControlDevRef"=w406) -> ()  [unwired: 7 in, 3 out]
          }
          frame True {
            n194 = call <vilib>:"WPI_MotorControlSetOutput.vi"("Output"=-0.15, "MotorControlDevRef"=w408) -> ()  [unwired: 7 in, 3 out]
          }
        }
      }
    }
    n195 = case shown="False" w376 {
      tunnel: w375 -> [_ w393]
      tunnel: w374 -> [_ w392]
      frame False {
      }
      frame True {
        n196 = call <vilib>:"WPI_EncoderReset.vi"("error in (no error)"=w392, "EncoderDevRef"=w393) -> ()  [unwired: 8 in, 2 out]
      }
    }
    n197 = Wait (ms)(milliseconds to wait=u32 50) -> ()  [unwired: 1 out]
  }
  n198 = call <vilib>:"WPI_ServoRefNum Registry Get.vi"("refnum name"="Actuator") -> ("ServoDeviceRef"=w12:T15)  [unwired: 9 in, 1 out]
  n199 = call <vilib>:"WPI_MotorControlRefNum Registry Get.vi"("refnum name"="Shooter Fire") -> ("error out"=w14:errorcluster, "MotorControlDevRef"=w15:T4)  [unwired: 9 in]
  n200 = call <vilib>:"WPI_MotorControlRefNum Registry Get.vi"("refnum name"="Shooter") -> ("error out"=w16:errorcluster, "MotorControlDevRef"=w17:T4)  [unwired: 9 in]
  n201 = while {
    tunnel: w17 -> [w422]
    tunnel: w16 -> [w421]
    tunnel: w15 -> [w416]
    tunnel: w14 -> [w415]
    tunnel: w12 -> [w419]
    stop <- FALSE stop-if-true
    # "100 ms tasks go here"
    n202 = Wait (ms)(milliseconds to wait=u32 50) -> ()  [unwired: 1 out]
    n203 = call-poly <vilib>:"NT Read Value.vi"("Name"="Shooter Height") -> ("Numeric"=w417:dbl)  [unwired: 9 in, 1 out]
    n204 = call-poly <vilib>:"NT Read Value.vi"("Name"="DB/FIRE SPD") -> ("Numeric"=w410:dbl)  [unwired: 9 in, 1 out]
    n205 = call-poly <vilib>:"NT Read Value.vi"("Name"="Shooter Fire") -> ("Boolean"=w414:bool)  [unwired: 9 in, 1 out]
    n206 = call-poly <vilib>:"NT Read Value.vi"("Name"="Shooter Inv") -> ("Boolean"=w412:bool)  [unwired: 9 in, 1 out]
    n207 = call-poly <vilib>:"NT Read Value.vi"("Name"="Shooter") -> ("Boolean"=w423:bool)  [unwired: 9 in, 1 out]
    n208 = call <vilib>:"WPI_ServoSetPosition.vi"("Position"=w417, "ServoDeviceRef"=w419) -> ()  [unwired: 8 in, 2 out]
    n209 = case shown="True" w423 {
      tunnel: w422 -> [w455 w460]
      tunnel: w421 -> [w454 w459]
      frame False {
        n210 = call <vilib>:"WPI_MotorControlSetOutput.vi"("error in (no error)"=w454, "Output"=0.0, "MotorControlDevRef"=w455) -> ()  [unwired: 6 in, 3 out]
      }
      frame True {
        n211 = call-poly <vilib>:"NT Read Value.vi"("Name"="Shooter Speed") -> ("Numeric"=w457:dbl)  [unwired: 9 in, 1 out]
        n212 = call <vilib>:"WPI_MotorControlSetOutput.vi"("error in (no error)"=w459, "Output"=w457, "MotorControlDevRef"=w460) -> ()  [unwired: 6 in, 3 out]
      }
    }
    n213 = case shown="False" w412 {
      tunnel: w416 -> [w429 w447]
      tunnel: w415 -> [w428 w446]
      tunnel: w414 -> [_ w445]
      tunnel: w410 -> [w427 w444]
      frame True {
        n214 = while {
          tunnel: w429 -> [w435]
          tunnel: w428 -> [w434]
          tunnel: w427 -> [w432]
          i -> [w440]
          stop <- w437 stop-if-true
          n215 = Multiply(x=w432, y=-0.5) -> (x*y=w431:dbl)
          n216 = call <vilib>:"WPI_MotorControlSetOutput.vi"("error in (no error)"=w434, "Output"=w431, "MotorControlDevRef"=w435) -> ()  [unwired: 6 in, 3 out]
          n217 = Greater?(x=2, y=3) -> (0:w436:bool)
          n218 = Greater?(x=w440, y=4) -> (0:w437:bool)
          n219 = case shown="True" w436 {
            frame False {
            }
            frame True {
              n220 = call-poly <vilib>:"NT Write Value.vi"("Boolean"=FALSE, "Name"="Shooter Inv") -> ()  [unwired: 9 in, 1 out]
            }
          }
          n221 = Wait (ms)(milliseconds to wait=u32 50) -> ()  [unwired: 1 out]
        }
      }
      frame False {
        n222 = case shown="True" w445 {
          tunnel: w447 -> [w449 w453]
          tunnel: w446 -> [w448 w452]
          tunnel: w444 -> [_ w451]
          frame False {
            n223 = call <vilib>:"WPI_MotorControlSetOutput.vi"("error in (no error)"=w448, "Output"=0.0, "MotorControlDevRef"=w449) -> ()  [unwired: 6 in, 3 out]
          }
          frame True {
            n224 = call <vilib>:"WPI_MotorControlSetOutput.vi"("error in (no error)"=w452, "Output"=w451, "MotorControlDevRef"=w453) -> ()  [unwired: 6 in, 3 out]
          }
        }
      }
    }
  }
  n225 = disable-structure shown="Disabled" {
    frame Disabled {
      n226 = call <vilib>:"WPI_SwitchRefNum Registry Get.vi"("refnum name"="CW Up") -> ("error out"=w461:errorcluster, "SwitchDevRef"=w462:T13)  [unwired: 9 in]
      n227 = call <vilib>:"WPI_MotorControlRefNum Registry Get.vi"("refnum name"="CW Drive") -> ("MotorControlDevRef"=w464:T4)  [unwired: 9 in, 1 out]
      n228 = call <vilib>:"Color Sensor V3 RefNum Registry Get.vi"("refnum name"="Color") -> ("ColorSensorDevRef"=w466:T10)  [unwired: 9 in, 1 out]
      n229 = while {
        tunnel: w466 -> [w479]
        tunnel: w464 -> [w470]
        tunnel: w462 -> [w477]
        tunnel: w461 -> [w476]
        stop <- FALSE stop-if-true
        # "100 ms tasks go here"
        n230 = call <vilib>:"Color Sensor V3 Get Color.vi"("ColorSensorDevRef"=w479) -> ("Normalized Color"=w478:cluster{"R":dbl, "G":dbl, "B":dbl})  [unwired: 7 in, 3 out]
        n231 = call <vilib>:"Color Sensor V3 Match Color.vi"("Measured Color"=w478) -> ("Matched Color Name"=w471:string)  [unwired: 8 in, 2 out]
        n232 = call <vilib>:"WPI_SwitchGetLimitValue.vi"("error in (no error)"=w476, "SwitchDevRef"=w477) -> ("Switch Pressed"=w473:bool)  [unwired: 7 in, 2 out]
        n233 = Wait (ms)(milliseconds to wait=u32 50) -> ()  [unwired: 1 out]
        n234 = call-poly <vilib>:"NT Write Value.vi"("String"=w471, "Name"="Color") -> ()  [unwired: 9 in, 1 out]
        n235 = call-poly <vilib>:"NT Read Value.vi"("Name"="Color Wheel ") -> ("String"=w472:string)  [unwired: 9 in, 1 out]
        n236 = case shown="True" w473 {
          tunnel: w472 -> [_ w484]
          tunnel: w471 -> [_ w483]
          tunnel: w470 -> [_ w482]
          frame False {
          }
          frame True {
            n237 = case shown="Default" w484 {
              tunnel: w483 -> [w488 w493 w502 w510 _ _ _]
              tunnel: w482 -> [w486 w494 w501 w509 w517 w520 w521]
              frame "Red" {
                n238 = Equal?(x=w488, y="Blue") -> (x = y?=w487:bool)
                n239 = case shown="False" w487 {
                  tunnel: w486 -> [w490 w492]
                  frame False {
                    n240 = call <vilib>:"WPI_MotorControlSetOutput.vi"("Output"=0.1, "MotorControlDevRef"=w490) -> ()  [unwired: 7 in, 3 out]
                  }
                  frame True {
                    n241 = call <vilib>:"WPI_MotorControlSetOutput.vi"("Output"=0.0, "MotorControlDevRef"=w492) -> ()  [unwired: 7 in, 3 out]
                  }
                }
              }
              frame "Yellow" {
                n242 = Equal?(x=w493, y="Green") -> (x = y?=w496:bool)
                n243 = case shown="False" w496 {
                  tunnel: w494 -> [w498 w500]
                  frame False {
                    n244 = call <vilib>:"WPI_MotorControlSetOutput.vi"("Output"=0.1, "MotorControlDevRef"=w498) -> ()  [unwired: 7 in, 3 out]
                  }
                  frame True {
                    n245 = call <vilib>:"WPI_MotorControlSetOutput.vi"("Output"=0.0, "MotorControlDevRef"=w500) -> ()  [unwired: 7 in, 3 out]
                  }
                }
              }
              frame "Green" {
                n246 = Equal?(x=w502, y="Yellow") -> (x = y?=w504:bool)
                n247 = case shown="False" w504 {
                  tunnel: w501 -> [w506 w508]
                  frame False {
                    n248 = call <vilib>:"WPI_MotorControlSetOutput.vi"("Output"=0.1, "MotorControlDevRef"=w506) -> ()  [unwired: 7 in, 3 out]
                  }
                  frame True {
                    n249 = call <vilib>:"WPI_MotorControlSetOutput.vi"("Output"=0.0, "MotorControlDevRef"=w508) -> ()  [unwired: 7 in, 3 out]
                  }
                }
              }
              frame "Blue" {
                n250 = Equal?(x=w510, y="Red") -> (x = y?=w512:bool)
                n251 = case shown="True" w512 {
                  tunnel: w509 -> [w513 w515]
                  frame False {
                    n252 = call <vilib>:"WPI_MotorControlSetOutput.vi"("Output"=0.1, "MotorControlDevRef"=w513) -> ()  [unwired: 7 in, 3 out]
                  }
                  frame True {
                    n253 = call <vilib>:"WPI_MotorControlSetOutput.vi"("Output"=0.0, "MotorControlDevRef"=w515) -> ()  [unwired: 7 in, 3 out]
                  }
                }
              }
              frame "Rotation" {
                n254 = call <vilib>:"WPI_MotorControlSetOutput.vi"("Output"=0.2, "MotorControlDevRef"=w517) -> ()  [unwired: 7 in, 3 out]
              }
              frame "Off" {
                n255 = call <vilib>:"WPI_MotorControlSetOutput.vi"("Output"=0.0, "MotorControlDevRef"=w520) -> ()  [unwired: 7 in, 3 out]
              }
              frame Default {
                n256 = call <vilib>:"WPI_MotorControlSetOutput.vi"("Output"=0.0, "MotorControlDevRef"=w521) -> ()  [unwired: 7 in, 3 out]
              }
            }
          }
        }
      }
      n257 = case shown="False" {
        selector: _ -> [_ _]
        frame False {
          n258 = call <vilib>:"WPI_MotorControlSetOutput.vi"("Output"=0.0) -> ()  [unwired: 8 in, 3 out]
        }
        frame True {
          n259 = call <vilib>:"WPI_MotorControlSetOutput.vi"("Output"=0.0) -> ()  [unwired: 8 in, 3 out]
        }
      }
    }
    frame Enabled {
    }
  }
